vi "Deinitialize.vi"(8 "error in":errorcluster, 11 "task in":i32) -> (0 "error out":errorcluster)   [LabVIEW 2020, in "DO_Relay.lvlib"]
uses:
  DO_Relay.lvlib
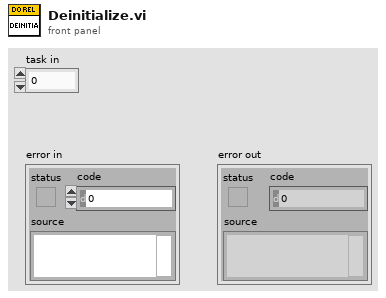
[diagram p1: front panel]
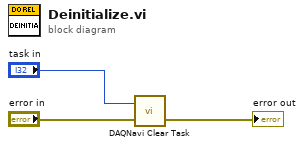
[diagram p0: block diagram]
diagram:
  n1 = call <userlib>:"DAQNavi Clear Task.vi"("error in (no error)"="error in", "task in"="task in") -> ("error out"=→"error out":errorcluster)  [unwired: 1 out]
